vi "COMMIT (ROLLBACK on Error).vi"(7 "Savepoint name":string caption="Savepoint to Release", 8 "error in (no error)":errorcluster, 11 "Connection in":refnum<class "Connection.lvclass">) -> (0 "error out":errorcluster, 3 "Connection out":refnum<class "Connection.lvclass">)   [LabVIEW 2013, in "SQLiteSupport.lvlib" / "Transaction.lvlib"]
doc: "COMMIT a transaction, or RELEASE the named Savepoint. Any nested Savepoints will also be released.\n\nOn an input <b>Error</b>, the transaction or Savepoint will instead be <b>rolled back</b> (ROLLBACK)."
uses:
  Transaction.lvlib
  SQL Connection/Connection.lvclass
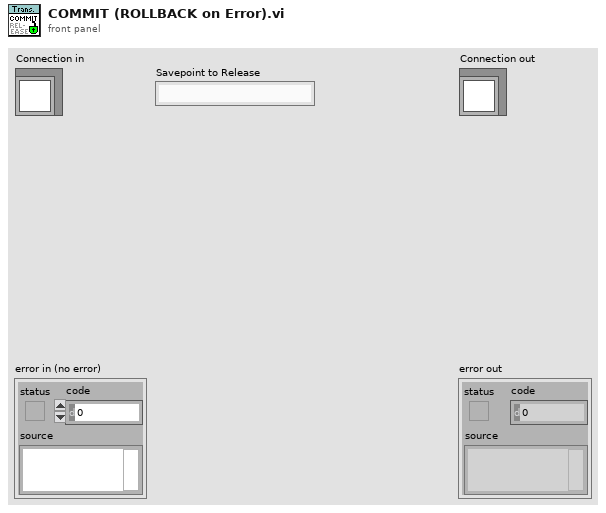
[diagram p1: front panel]
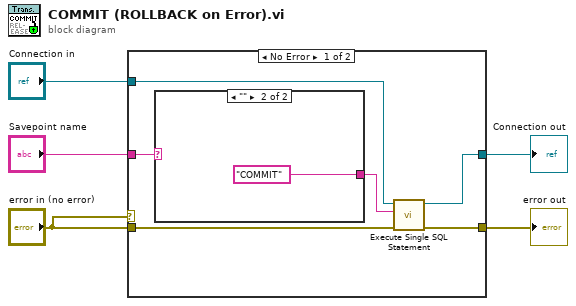
[diagram p0: block diagram]
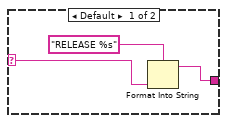
[diagram p2: hidden frame]
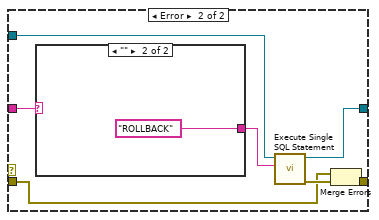
[diagram p3: hidden frame]
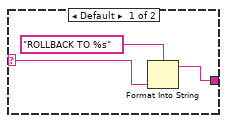
[diagram p4: hidden frame]
diagram:
  n1 = case shown="No Error" "error in (no error)" {
    tunnel: "error in (no error)" -> [w11 w16]
    tunnel: [w10 w17] -> w5
    tunnel: "Connection in" -> [w9 w21]
    tunnel: [w8 w20] -> w3
    tunnel: "Savepoint name" -> [w7 w19]
    frame No Error {
      n2 = case shown="\"\"" w7 {
        selector: w7 -> [w14 _]
        tunnel: [w12 "COMMIT"] -> w6
        frame Default {
          n3 = Format Into String(format string="RELEASE %s", w14) -> (resulting string=w12:string)  [unwired: 2 in, 1 out]
        }
        frame "" {
        }
      }
      n4 = call "Execute Single SQL Statement.vi"("error in (no error)"=w11, "SQL statement"=w6, "SQLite Connection in"=w9) -> ("error out"=w10:errorcluster, "SQLite Connection out"=w8:refnum<class "Connection.lvclass">)  [unwired: 7 in]
    }
    frame Error {
      n5 = case shown="\"\"" w19 {
        selector: w19 -> [w25 _]
        tunnel: [w23 "ROLLBACK"] -> w18
        frame Default {
          n6 = Format Into String(format string="ROLLBACK TO %s", w25) -> (resulting string=w23:string)  [unwired: 2 in, 1 out]
        }
        frame "" {
        }
      }
      n7 = call "Execute Single SQL Statement.vi"("SQL statement"=w18, "SQLite Connection in"=w21) -> ("error out"=w22:errorcluster, "SQLite Connection out"=w20:refnum<class "Connection.lvclass">)  [unwired: 8 in]
      n8 = Merge Errors(w16, w22) -> (w17:errorcluster)
    }
  }
  "error out" <- w5
  "Connection out" <- w3
